vi "F15.vi"(8 "error in":errorcluster, 9 "data":u8[](array[numeric]), 10 "function":u8, 11 "device data model in":refnum<class "Standard Data Model.lvclass">) -> (0 "error out":errorcluster, 1 "data return":u8[](array[numeric]), 2 "function return":u8, 3 "device data model out":refnum<class "Standard Data Model.lvclass">)   [LabVIEW 2012, in "Standard Data Model.lvclass"]
doc: "Executes function code 15"
uses:
  Standard Data Model.lvclass
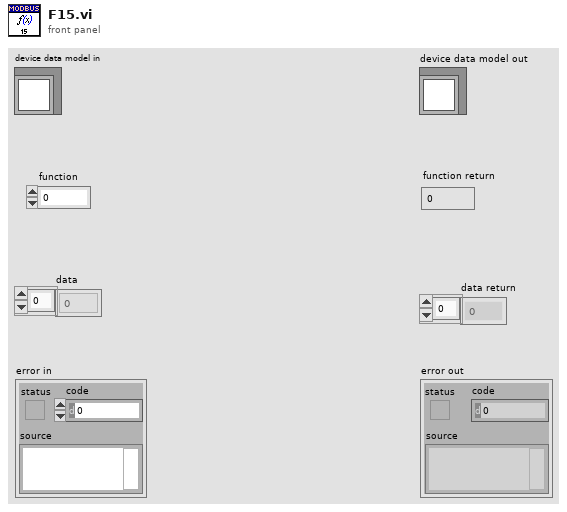
[diagram p1: front panel]
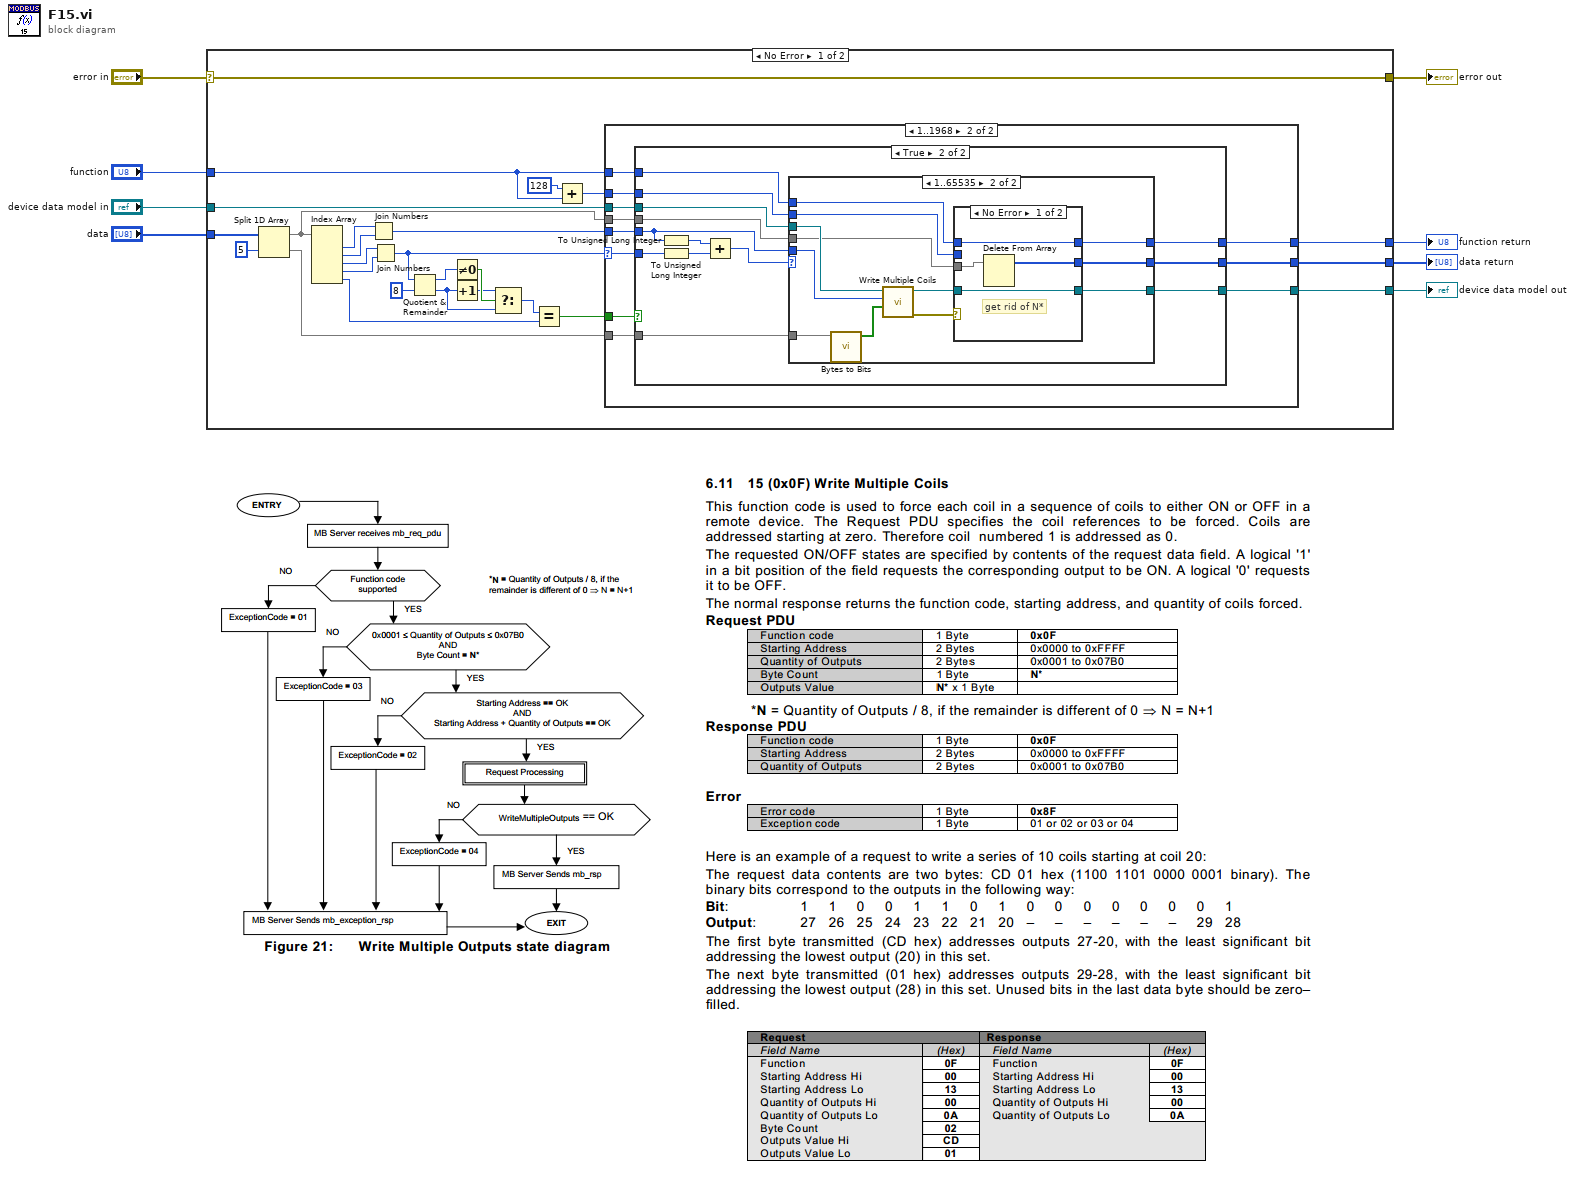
[diagram p0: block diagram]
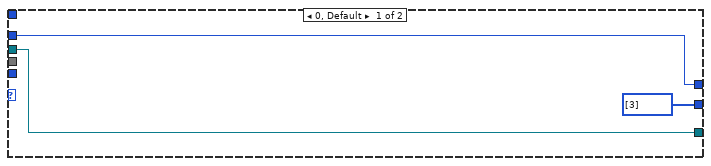
[diagram p2: hidden frame]
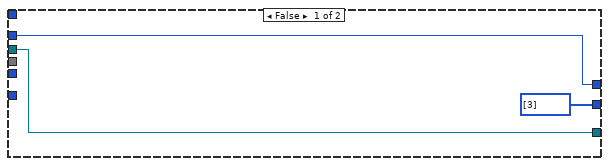
[diagram p3: hidden frame]
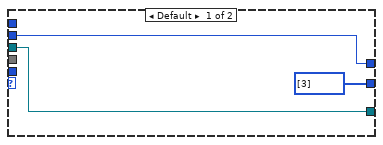
[diagram p4: hidden frame]
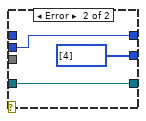
[diagram p5: hidden frame]
diagram:
  n1 = case shown="No Error" "error in" {
    selector: "error in" -> [w21 w90]
    tunnel: [w21 w90] -> w7
    tunnel: [w34 w89] -> w5
    tunnel: "device data model in" -> [w33 w89]
    tunnel: "function" -> [w30 w88]
    tunnel: "data" -> [w27 w87]
    tunnel: [w29 w88] -> w2
    tunnel: [w28 w87] -> w1
    frame No Error {
      n2 = Split 1D Array(array=w27, index=5) -> (first subarray=w22:u8[], second subarray=w25:u8[])
      n3 = Index Array(array=w22) -> (element #1=w19:u8, element #2=w20:u8, element #3=w24:u8, element #4=w23:u8, element #5=w10:u8)  [unwired: 5 in]
      n4 = Join Numbers(hi=w19, lo=w20) -> ((hi.lo)=w18:u16)
      n5 = Join Numbers(hi=w24, lo=w23) -> ((hi.lo)=w12:u16)
      n6 = Quotient & Remainder(x=w12, y=u16 8) -> (x-y*floor(x/y)=w15:u16, floor(x/y)=w9:u16)
      n7 = Not Equal To 0?(x=w15) -> (x != 0?=w17:bool)
      n8 = Increment(x=w9) -> (x+1=w16:u16)
      n9 = Select(t=w16, s=w17, f=w9) -> (s? t:f=w11:u16)
      n10 = Equal?(x=w11, y=w10) -> (x = y?=w14:bool)
      n11 = Add(x=u8 128, y=w30) -> (x+y=w31:u8)
      n12 = case shown="1..1968" w12 {
        selector: w12 -> [_ w38]
        tunnel: [w35 w48] -> w34
        tunnel: w33 -> [w35 w47]
        tunnel: w31 -> [w37 w46]
        tunnel: w30 -> [_ w45]
        tunnel: [w37 w44] -> w29
        tunnel: [u8[] [3] ("Data Return") w43] -> w28
        tunnel: w25 -> [_ w42]
        tunnel: w22 -> [_ w41]
        tunnel: w18 -> [_ w40]
        tunnel: w14 -> [_ w39]
        frame 0, Default {
        }
        frame 1..1968 {
          n13 = case shown="True" w39 {
            tunnel: [w49 w64] -> w48
            tunnel: w47 -> [w49 w58]
            tunnel: w46 -> [w50 w63]
            tunnel: w45 -> [_ w62]
            tunnel: [w50 w61] -> w44
            tunnel: [u8[] [3] ("Data Return") w60] -> w43
            tunnel: w42 -> [_ w59]
            tunnel: w38 -> [_ w53]
            tunnel: w41 -> [_ w57]
            tunnel: w40 -> [_ w54]
            frame False {
            }
            frame True {
              n14 = To Unsigned Long Integer(number=w54) -> (unsigned 32bit integer=w55:u32)
              n15 = To Unsigned Long Integer(number=w53) -> (unsigned 32bit integer=w52:u32)
              n16 = Add(x=w55, y=w52) -> (x+y=w56:u32)
              n17 = case shown="1..65535" w56 {
                tunnel: [w67 w79] -> w64
                tunnel: w58 -> [w67 w74]
                tunnel: w63 -> [w66 w78]
                tunnel: w62 -> [_ w76]
                tunnel: [w66 w77] -> w61
                tunnel: [u8[] [3] ("Data Return") w75] -> w60
                tunnel: w59 -> [_ w69]
                tunnel: w57 -> [_ w73]
                tunnel: w54 -> [_ w70]
                frame Default {
                }
                frame 1..65535 {
                  n18 = call "Bytes to Bits.vi"("Bytes"=w69) -> ("Bits"=w68:bool[])  [unwired: 10 in]
                  n19 = call-dynamic "Write Multiple Coils.vi"("coils"=w68, "starting address"=w70, "device data model in"=w74) -> ("error out"=w72:errorcluster, "device data model out"=w71:refnum<class "Standard Data Model.lvclass">)  [unwired: 7 in]
                  n20 = case shown="No Error" w72 {
                    tunnel: w71 -> [w83 w86]
                    tunnel: [w83 w86] -> w79
                    tunnel: w78 -> [_ w85]
                    tunnel: w76 -> [w82 _]
                    tunnel: [w82 w85] -> w77
                    tunnel: [w80 u8[] [4]] -> w75
                    tunnel: w73 -> [w81 _]
                    frame No Error {
                      # "get rid of N*"
                      n21 = Delete From Array(array=w81) -> (array with subset deleted=w80:u8[])  [unwired: 2 in, 1 out]
                    }
                    frame Error {
                    }
                  }
                }
              }
            }
          }
        }
      }
    }
    frame Error {
    }
  }
  "error out" <- w7
  "device data model out" <- w5
  "data return" <- w1
  "function return" <- w2
